vi "IntakeExecute.vi"(8 "error in (no error)":errorcluster) -> (0 "error out":errorcluster)   [LabVIEW 2023]
uses:
  <vilib>/Rock Robotics/WPI/ThirdParty/JAS_Junk/TrajLib/VI/BoolCmd_Recv.vi
  <vilib>/Rock Robotics/WPI/ThirdParty/JAS_Junk/TrajLib/VI/BoolCmd_Multiplexor_Array.vi
  IntakeStateMachine.vi
  <vilib>/Rock Robotics/WPI/ThirdParty/JAS_Junk/TrajLib/VI/BoolCmd_Recv_Internal.vi
  <vilib>/Rock Robotics/WPI/ThirdParty/JAS_Junk/TrajLib/VI/DigSeqLogic_Edge_On.vi
  <vilib>/Rock Robotics/WPI/ThirdParty/JAS_Junk/TrajLib/VI/BoolCmd_ObtainQueue.vi
  IntakeGlobal.vi
panel:
  # "Click here to set min"
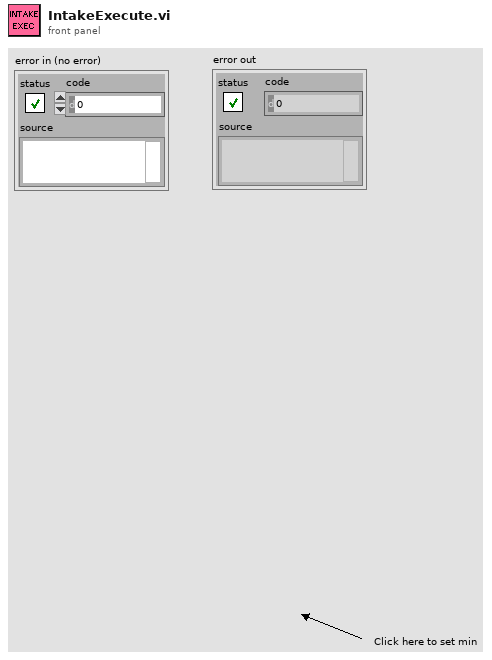
[diagram p1: front panel]
types:
  T1 = typedef "WPI_MotorControlDeviceRef.ctl" = cluster{"DeviceStatus":errorcluster, "Type":T2, "PWM":cluster{"PWM Channel":T3, "DeadBand":T4}, "CAN":cluster{"Device Number":u8, "SetOutput VI Ref":variant, "GetOutput VI Ref":variant, "Enable VI Ref":variant, "Disable VI Ref":variant, "Data":variant}, "Invert":bool, "DIO PWM":cluster{"PWM \"Enable\" Channel":T3, "DIOChannel":T5, "PWM Rate":dbl}}
  T2 = typedef "WPI_MotorControlType.ctl" = enum16{"PWM", "CAN", "DIO PWM"}
  T3 = typedef "FPGA_DIOPWMChannel.ctl" = enum8{"PWM 0", "PWM 1", "PWM 2", "PWM 3", "PWM 4", "PWM 5", "PWM 6", "PWM 7", "PWM 8", "PWM 9", "PWM MXP 0", "PWM MXP 1", "PWM MXP 2", "PWM MXP 3", "PWM MXP 4", "PWM MXP 5", "PWM MXP 6", "PWM MXP 7", "PWM MXP 8", "PWM MXP 9", "Invalid"}
  T4 = typedef "WPI_PWMDeadband.ctl" = cluster{"Name":string, "maxPositivePwm":i32, "minPositivePwm":i32, "centerPwm":i32, "maxNegativePwm":i32, "minNegativePwm":i32, "angularRange":u16}
  T5 = typedef "FPGA_DIOChannel.ctl" = enum8{"DIO 0", "DIO 1", "DIO 2", "DIO 3", "DIO 4", "DIO 5", "DIO 6", "DIO 7", "DIO 8", "DIO 9", "DIO MXP 0", "DIO MXP 1", "DIO MXP 2", "DIO MXP 3", "DIO MXP 4", "DIO MXP 5", "DIO MXP 6", "DIO MXP 7", "DIO MXP 8", "DIO MXP 9", "DIO MXP 10", "DIO MXP 11", "DIO MXP 12", "DIO MXP 13", "DIO MXP 14", "DIO MXP 15", "SPI Port CS1", "SPI Port CS2", "SPI Port CS3", "SPI Port MISO", "SPI Port MOSI", "Invalid"}
  T6 = typedef "WPI_SwitchDevRef.ctl" = cluster{"DevStatus":errorcluster, "DIO Channel":T5, "CntIndex":T7, "Normally Closed":bool}
  T7 = typedef "FPGA_CounterCtrSystemIndex.ctl" = enum8{"Ctr 0", "Ctr 1", "Ctr 2", "Ctr 3", "Ctr 4", "Ctr 5", "Ctr 6", "Ctr 7", "Invalid"}
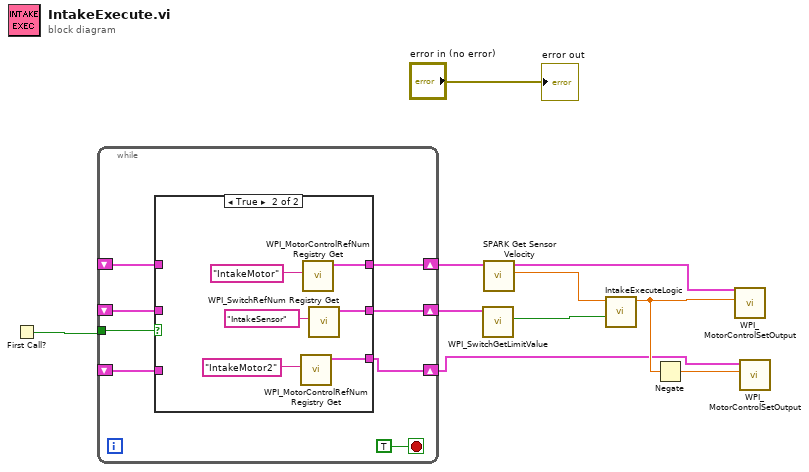
[diagram p0: block diagram]
diagram:
  n1 = First Call?() -> (First Call?: T/F=w8:bool)
  n2 = while {
    tunnel: w8 -> [w17]
    shift-right: [w18] -> w10
    shift-left: _ -> [w16]
    shift-right: [w14] -> w7
    shift-left: _ -> [w13]
    shift-right: [w12] -> w1
    shift-left: _ -> [w11]
    stop <- TRUE stop-if-true
    n3 = case shown="True" w17 {
      tunnel: [w21 w27] -> w18
      tunnel: w16 -> [w21 _]
      tunnel: [w20 w24] -> w14
      tunnel: w13 -> [w20 _]
      tunnel: [w19 w22] -> w12
      tunnel: w11 -> [w19 _]
      frame False {
      }
      frame True {
        n4 = call <vilib>:"WPI_MotorControlRefNum Registry Get.vi"("refnum name"="IntakeMotor2") -> ("MotorControlDevRef"=w22:T1)  [unwired: 9 in, 1 out]
        n5 = call <vilib>:"WPI_MotorControlRefNum Registry Get.vi"("refnum name"="IntakeMotor") -> ("MotorControlDevRef"=w24:T1)  [unwired: 9 in, 1 out]
        n6 = call <vilib>:"WPI_SwitchRefNum Registry Get.vi"("refnum name"="IntakeSensor") -> ("SwitchDevRef"=w27:T6)  [unwired: 9 in, 1 out]
      }
    }
  }
  n7 = call <vilib>:"WPI_SwitchGetLimitValue.vi"("SwitchDevRef"=w10) -> ("Switch Pressed"=w4:bool)  [unwired: 8 in, 2 out]
  n8 = call <vilib>:"SPARK Get Sensor Velocity.vi"("MotorControlDevRef in"=w7) -> ("Sensor Velocity"=w5:dbl, "MotorControlDevRef out"=w6:T1)  [unwired: 7 in, 2 out]
  n9 = call "IntakeExecuteLogic.vi"("HaveNoteSensor"=w4, "Sensor Velocity"=w5) -> ("MotorOutDmd"=w3:dbl)  [unwired: 9 in]
  n10 = Negate(x=w3) -> (-x=w2:dbl)
  n11 = call <vilib>:"WPI_MotorControlSetOutput.vi"("Output"=w3, "MotorControlDevRef"=w6) -> ()  [unwired: 7 in, 3 out]
  n12 = call <vilib>:"WPI_MotorControlSetOutput.vi"("Output"=w2, "MotorControlDevRef"=w1) -> ()  [unwired: 7 in, 3 out]
  "error out" <- "error in (no error)"
